vi "Kill Loader.vi"(10 "Log":bool=TRUE, 11 "PIDs":u32[](array[numeric])) -> (0 "error out":errorcluster, 2 "Failed to stop":bool, 3 "Kill Action":T1(ring))   [LabVIEW 2021, in "CIFPluginManager.lvclass"]
uses:
  CIFPluginManager.lvclass
  typedef/Kill Statemachine.ctl
  CIFCore/Common/Typedef/Errors.ctl
  CIFUtilities/CIFLogs/Typedef/Message Type.ctl
  <vilib>/CIF Foundation/CIF Utilities/Errors/Append Error Location.vi
  CIFPluginManager.lvclass/CIFPluginManager.ctl
  CIFUtilities/CIFLogs/CIFLogs.lvlib
  CIFCore/Common/CIFCoreCommon.lvlib
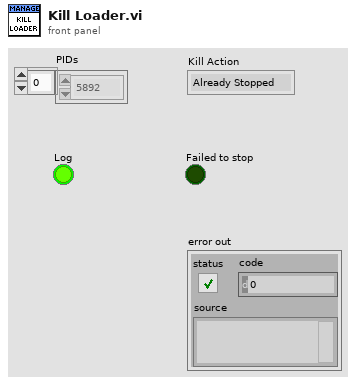
[diagram p1: front panel]
types:
  T1 = enum16{"Already Stopped", "SigInt", "SigTerm", "SigKill"}
  T2 = typedef "CIFCoreCommon.lvlib/Errors.ctl" = enum16{"Invalid Clock ID", "Long Sleep", "gRPC Server Not Found", "Config Parse", "Timestamp Wrap", "Delayed Execution", "Duplicate Channel", "Missing Channel", "Incorrect Type", "Flatten Error", "Unflatten Data", "Unique Name", "Plugin Not Found", "Plugin Type Not Found", "Plugin Version Not Found", "Manager Not Found", "Numerical Issue", "Time Jump", "Clock ID Match", "Channel Length", "Plugin Connection", "gRPC Server Connection", "PPL Name Match", "Build", "Config Log Parse", "Plugin Load", "UI Subpanel Load", "Python Name", "Invalid Name", "Unable to Change Ch Buffer", "Failed Kill"}
  T3 = typedef "CIFPluginManager.lvclass/Kill Statemachine.ctl" = enum16{"Check for Running", "Sleep", "SigInt", "SigTerm", "SigKill"}
  T4 = typedef "CIFLogs.lvlib/Message Type.ctl" = enum16{"Error", "Information", "Print Terminal", "Configuration"}
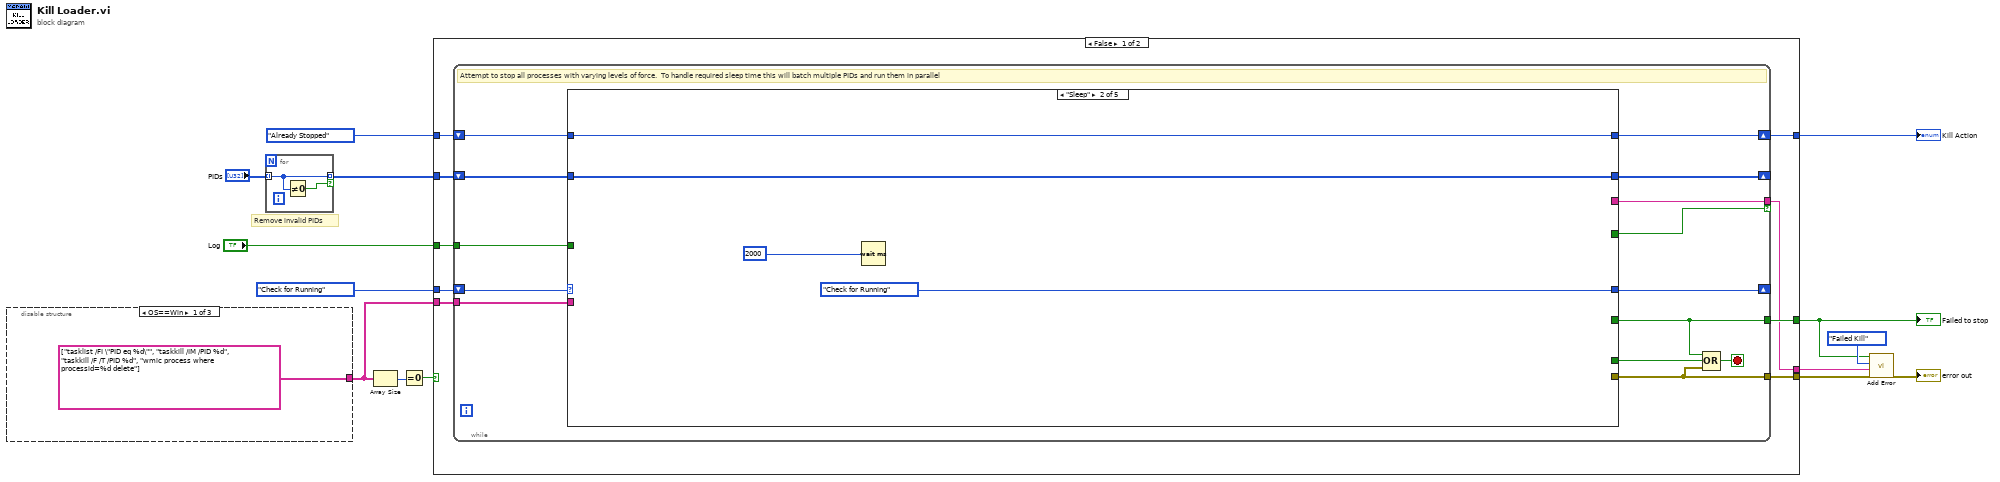
[diagram p0: block diagram]
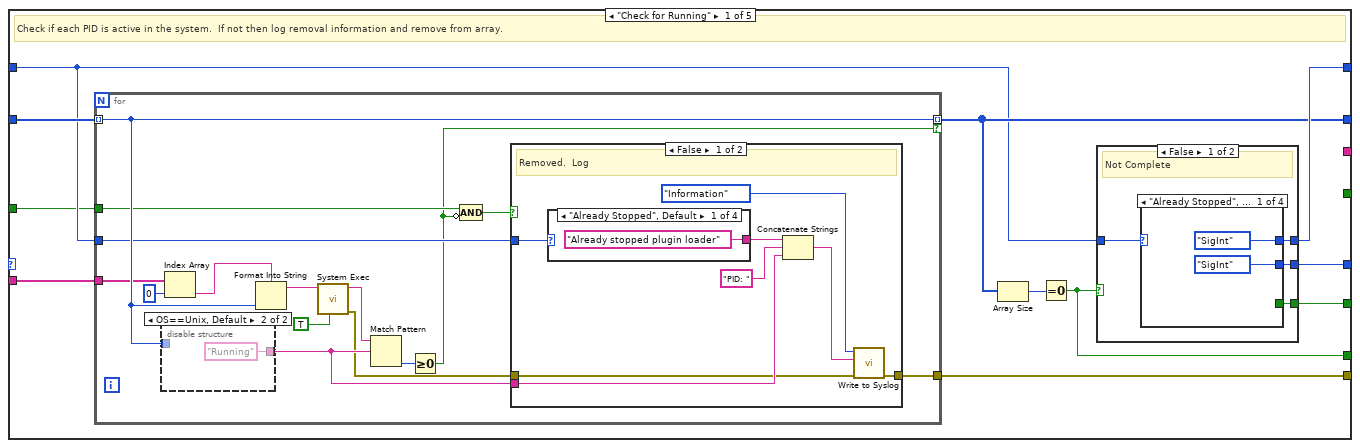
[diagram p2: hidden frame]
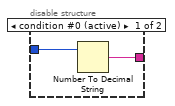
[diagram p3: hidden frame]
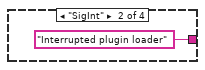
[diagram p4: hidden frame]
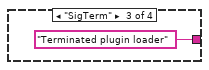
[diagram p5: hidden frame]
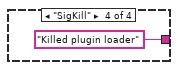
[diagram p6: hidden frame]
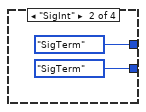
[diagram p8: hidden frame]
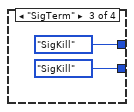
[diagram p9: hidden frame]
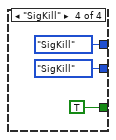
[diagram p10: hidden frame]
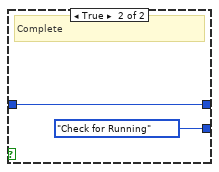
[diagram p11: hidden frame]
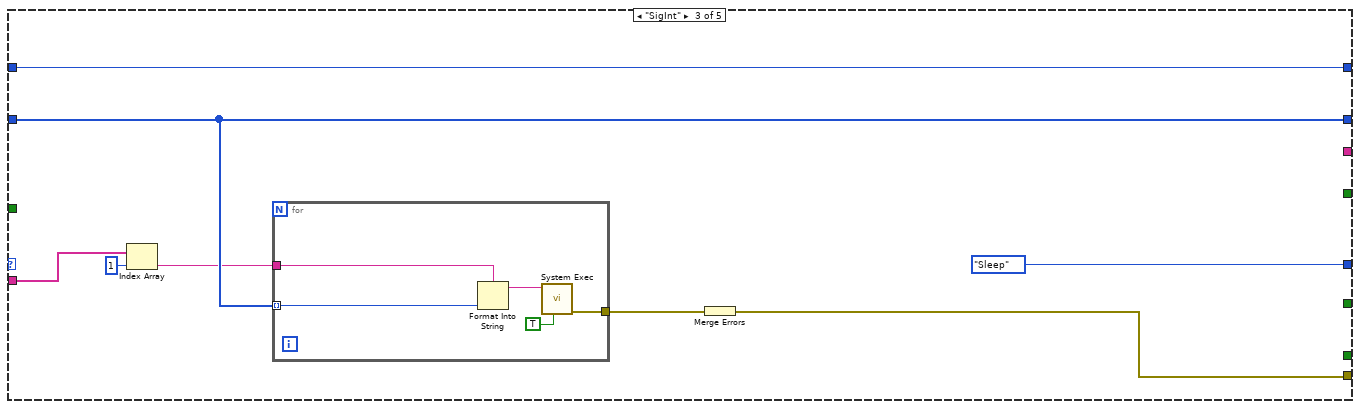
[diagram p12: hidden frame]
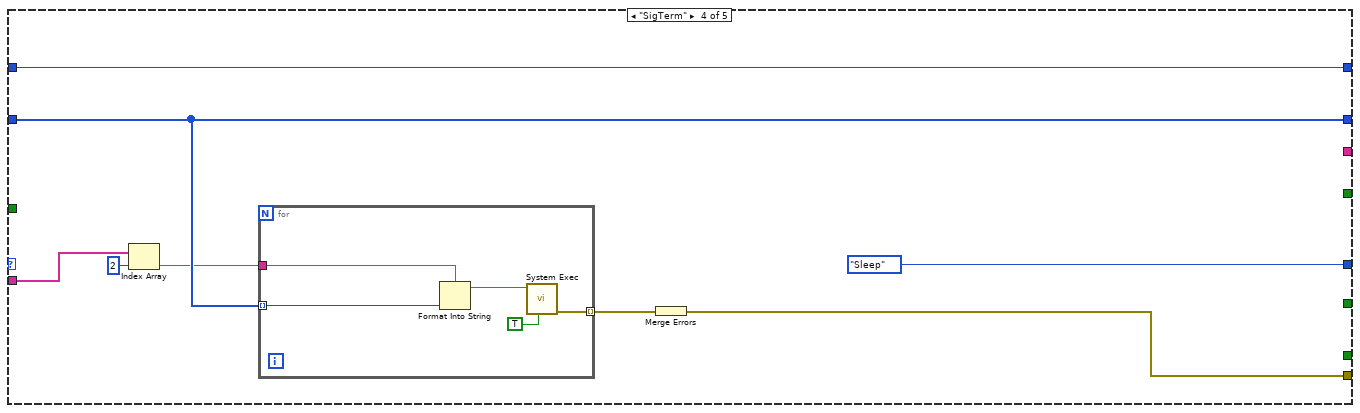
[diagram p13: hidden frame]
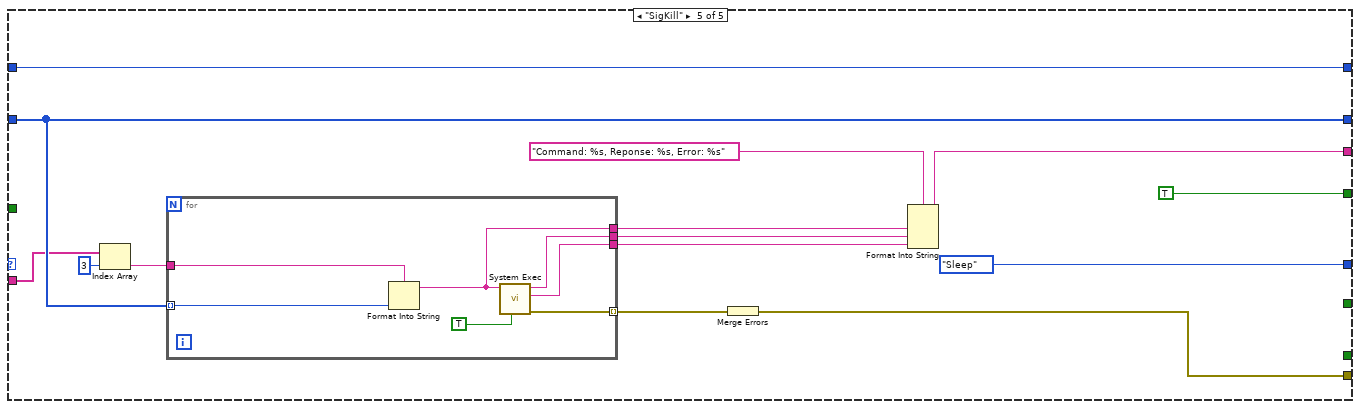
[diagram p14: hidden frame]
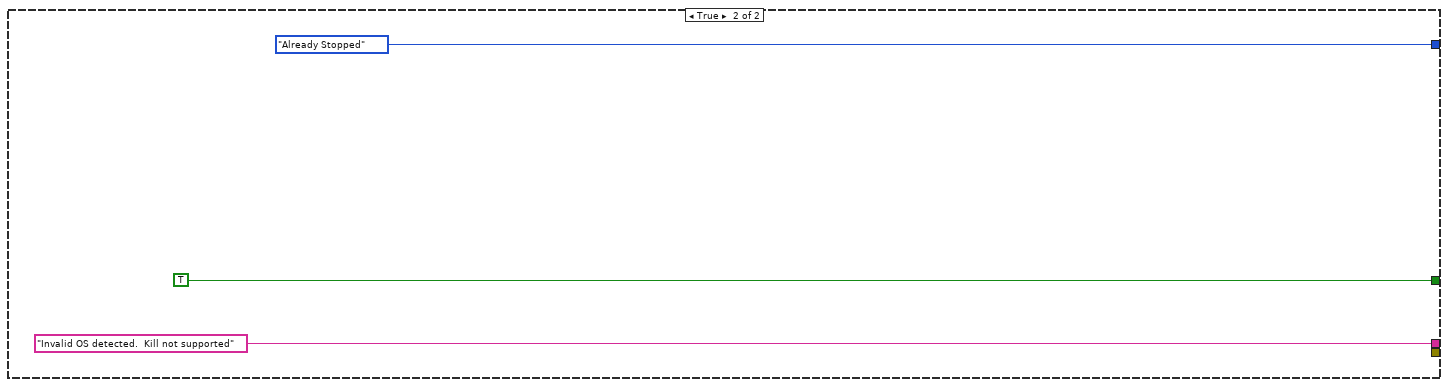
[diagram p15: hidden frame]
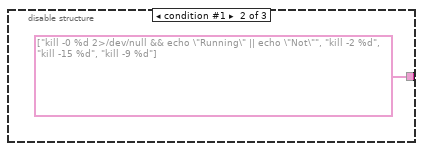
[diagram p16: hidden frame]
diagram:
  # "Remove invalid PIDs"
  n1 = disable-structure shown="OS==Win" {
    disable-tunnel: [string[] ["tasklist /FI \"PID eq %d\"", "taskkill /IM /PID %d", "taskkill /F /T /PID %d", "wmic process where processid=%d delete"] string[] ["kill -0 %d 2>/dev/null && echo \"Running\" || echo \"Not\"", "kill -2 %d", "kill -15 %d", "kill -9 %d"] _] -> w3
    frame condition #0 (active) {
    }
    frame condition #1 {
    }
    frame condition #2 {
    }
  }
  n2 = for {
    tunnel: "PIDs" -> [w18] mode=indexing
    tunnel: [w18] -> w10 mode=indexing if=w17
    n3 = Not Equal To 0?(x=w18) -> (x != 0?=w17:bool)
  }
  n4 = Array Size(array=w3) -> (size(s)=w4:i32)
  n5 = Equal To 0?(x=w4) -> (x = 0?=w1:bool)
  n6 = case shown="False" w1 {
    tunnel: Kill_Statemachine."Check for Running" ("Kill Statemachine") -> [w27 _]
    tunnel: T1."Already Stopped" ("Kill Result") -> [w26 _]
    tunnel: [w25 T1."Already Stopped" ("Kill Result")] -> w12
    tunnel: w10 -> [w24 _]
    tunnel: [w23 _] -> w8
    tunnel: [w22 TRUE] -> w2
    tunnel: [w21 "Invalid OS detected.  Kill not supported"] -> w6
    tunnel: "Log" -> [w20 _]
    tunnel: w3 -> [w19 _]
    frame False {
      n7 = while {
        shift-right: [w39] -> _
        shift-left: w27 -> [w41]
        shift-right: [w38] -> w25
        shift-left: w26 -> [w40]
        tunnel: [w31] -> w22
        tunnel: [w36] -> w21 if=w35
        tunnel: [w34] -> w23
        shift-right: [w32] -> _
        shift-left: w24 -> [w33]
        tunnel: w20 -> [w29]
        tunnel: w19 -> [w28]
        stop <- w37 stop-if-true
        # "Attempt to stop all processes with varying levels of force.  To handle required sleep time this will batch multiple PIDs and run them in parallel"
        n8 = case shown="\"Sleep\"" w41 {
          tunnel: [w45 _ _ _ _] -> w30
          tunnel: w40 -> [w44 w102 w110 w123 w142]
          tunnel: [w52 w102 w110 w123 w142] -> w38
          tunnel: [w51 Kill_Statemachine."Check for Running" ("Kill Statemachine") Kill_Statemachine."Sleep" ("Kill Statemachine") Kill_Statemachine."Sleep" ("Kill Statemachine") Kill_Statemachine."Sleep" ("Kill Statemachine")] -> w39
          tunnel: [w50 _ _ _ _] -> w31
          tunnel: [_ _ _ _ w136] -> w36
          tunnel: [_ _ _ _ TRUE] -> w35
          tunnel: [w49 _ w106 w120 w133] -> w34
          tunnel: w33 -> [w48 w99 w108 w119 w132]
          tunnel: [w46 w99 w108 w119 w132] -> w32
          tunnel: w29 -> [w43 _ _ _ _]
          tunnel: w28 -> [w42 _ w104 w116 w129]
          frame "Check for Running" {
            # "Check if each PID is active in the system.  If not then log removal information and remove from array."
            n9 = for {
              tunnel: [w59] -> w49
              tunnel: w48 -> [w63] mode=indexing
              tunnel: [w63] -> w46 mode=indexing if=w57
              tunnel: w44 -> [w61]
              tunnel: w43 -> [w58]
              tunnel: w42 -> [w55]
              n10 = disable-structure shown="OS==Unix, Default" {
                disable-tunnel: w63 -> [w69 _]
                disable-tunnel: [w68 "Running"] -> w62
                frame condition #0 (active) {
                  n11 = Number To Decimal String(number=w69) -> (decimal integer string=w68:string)  [unwired: 1 in]
                }
                frame condition #1 {
                }
              }
              n12 = Index Array(array=w55, index=0) -> (element=w54:string)
              n13 = Format Into String(format string=w54, w63) -> (resulting string=w67:string)  [unwired: 2 in, 1 out]
              n14 = call <vilib>:"System Exec.vi"("run minimized? (F)"=TRUE, "command line"=w67) -> ("error out"=w60:errorcluster, "standard output"=w65:string)  [unwired: 6 in, 2 out]
              n15 = Match Pattern(string=w65, regular expression=w62) -> (offset past match=w64:i32)  [unwired: 1 in, 3 out]
              n16 = Greater Or Equal To 0?(x=w64) -> (x >= 0?=w57:bool)
              n17 = Compound Arithmetic op=AND(w58, invert w57) -> (w56:bool)
              n18 = case shown="False" w56 {
                tunnel: w62 -> [w77 _]
                tunnel: w61 -> [w75 _]
                tunnel: w60 -> [w73 w83]
                tunnel: [w72 w83] -> w59
                frame False {
                  # "Removed.  Log"
                  n19 = case shown="\"Already Stopped\", Default" w75 {
                    tunnel: ["Already stopped plugin loader" ("message") "Interrupted plugin loader" ("message") "Terminated plugin loader" ("message") "Killed plugin loader" ("message")] -> w78
                    frame "Already Stopped", Default {
                    }
                    frame "SigInt" {
                    }
                    frame "SigTerm" {
                    }
                    frame "SigKill" {
                    }
                  }
                  n20 = Concatenate Strings(w78, "PID: " ("message"), w77) -> (w71:string)
                  n21 = call "Write to Syslog.vi"("error in (no error)"=w73, "message"=w71, "CIF Message Type"=Message_Type."Information") -> ("error out"=w72:errorcluster)  [unwired: 8 in]
                }
                frame True {
                  # "Not Removed"
                }
              }
            }
            n22 = Array Size(array=w46) -> (size(s)=w47:i32)
            n23 = Equal To 0?(x=w47) -> (x = 0?=w45:bool)
            n24 = case shown="False" w45 {
              tunnel: w44 -> [w87 w98]
              tunnel: [w85 w98] -> w52
              tunnel: [w86 Kill_Statemachine."Check for Running" ("Kill Statemachine")] -> w51
              tunnel: [w84 _] -> w50
              frame False {
                # "Not Complete"
                n25 = case shown="\"Already Stopped\", Default" w87 {
                  tunnel: [Kill_Statemachine."SigInt" ("Kill Statemachine") Kill_Statemachine."SigTerm" ("Kill Statemachine") Kill_Statemachine."SigKill" ("Kill Statemachine") Kill_Statemachine."SigKill" ("Kill Statemachine")] -> w86
                  tunnel: [T1."SigInt" ("Kill Result") T1."SigTerm" ("Kill Result") T1."SigKill" ("Kill Result") T1."SigKill" ("Kill Result")] -> w85
                  tunnel: [_ _ _ TRUE] -> w84
                  frame "Already Stopped", Default {
                  }
                  frame "SigInt" {
                  }
                  frame "SigTerm" {
                  }
                  frame "SigKill" {
                  }
                }
              }
              frame True {
                # "Complete"
              }
            }
          }
          frame "Sleep" {
            n26 = Wait (ms)(milliseconds to wait=u32 2000) -> ()  [unwired: 1 out]
          }
          frame "SigInt" {
            n27 = Index Array(array=w104, index=1) -> (element=w103:string)
            n28 = for {
              tunnel: w108 -> [w113] mode=indexing
              tunnel: [w112] -> w107
              tunnel: w103 -> [w111]
              n29 = Format Into String(format string=w111, w113) -> (resulting string=w115:string)  [unwired: 2 in, 1 out]
              n30 = call <vilib>:"System Exec.vi"("run minimized? (F)"=TRUE, "command line"=w115) -> ("error out"=w112:errorcluster)  [unwired: 6 in, 3 out]
            }
            n31 = Merge Errors(w107) -> (w106:errorcluster)
          }
          frame "SigTerm" {
            n32 = Index Array(array=w116, index=2) -> (element=w117:string)
            n33 = for {
              tunnel: w119 -> [w126] mode=indexing
              tunnel: [w125] -> w121 mode=indexing
              tunnel: w117 -> [w124]
              n34 = Format Into String(format string=w124, w126) -> (resulting string=w128:string)  [unwired: 2 in, 1 out]
              n35 = call <vilib>:"System Exec.vi"("run minimized? (F)"=TRUE, "command line"=w128) -> ("error out"=w125:errorcluster)  [unwired: 6 in, 3 out]
            }
            n36 = Merge Errors(w121) -> (w120:errorcluster)
          }
          frame "SigKill" {
            n37 = Index Array(array=w129, index=3) -> (element=w130:string)
            n38 = for {
              tunnel: w132 -> [w148] mode=indexing
              tunnel: [w147] -> w139
              tunnel: [w146] -> w138
              tunnel: [w145] -> w137
              tunnel: [w144] -> w134 mode=indexing
              tunnel: w130 -> [w143]
              n39 = Format Into String(format string=w143, w148) -> (resulting string=w147:string)  [unwired: 2 in, 1 out]
              n40 = call <vilib>:"System Exec.vi"("run minimized? (F)"=TRUE, "command line"=w147) -> ("error out"=w144:errorcluster, "standard error"=w145:string, "standard output"=w146:string)  [unwired: 6 in, 1 out]
            }
            n41 = Merge Errors(w134) -> (w133:errorcluster)
            n42 = Format Into String(format string="Command: %s, Reponse: %s, Error: %s" ("initial string"), w139, w138, w137) -> (resulting string=w136:string)  [unwired: 2 in, 1 out]
          }
        }
        n43 = Compound Arithmetic op=OR(w31, w30, w34) -> (w37:bool)
      }
    }
    frame True {
    }
  }
  "Failed to stop" <- w2
  "Kill Action" <- w12
  n44 = call "Add Error.vi"("error in (no error)"=w8, "String to Append"=w6, "Error"=Errors."Failed Kill", "Insert Error"=w2) -> ("error out"=→"error out":errorcluster)  [unwired: 7 in]
